vi "5.10 Occipital Lobei.vi"(9 "Randy":T3, 10 "Larry":T3) -> ()   [LabVIEW 2010]
uses:
  4-High Neurons/4.0-Timing Badass.ctl
  <vilib>/userDefined/High Color/IMAQdx.ctl
  5.10 Algorithm Parameters and Controls.ctl
  4-High Neurons/4.1.2-Act Neuron TD.ctl
  5.0-Global.vi
  <vilib>/vision/driver/NI_Vision_Acquisition_Software.lvlib
panel:
  in  "stop":bool
  out "Randy Steer Angle":dbl
  out "Larry Steer Angle":dbl
  out "Randy Certainty":dbl
  out "Larry Certainty":dbl
  in  "Rotation of Camera":dbl[][](array[numeric])=[[1.0, 0.0, 0.0], [0.0, 1.0, 0.0], [0.0, 0.0, 1.0]]
  in  "Location of Camera":dbl[](array[numeric])=[0.0, 0.0, 0.0]
  out "XY Graph":cluster{dbl[], dbl[]}[](graph)
  out "Randy Blue Actual":dbl
  out "Larry Blue Actual":dbl
  in  "Larry Exposure":dbl=0.02
  in  "Randy Exposure":dbl=0.02
  out "Randy B/W Overlay (R4)":T1(plugin-control)
  out "Randy Color Overlay (R5)":T1(plugin-control)
  in  "Randy Blue Threshold":i32=120
  out "Larry Color Overlay (L5)":T1(plugin-control)
  out "Larry B/W Overlay (L4)":T1(plugin-control)
  out "Larry Re-Map (L3)":T1(plugin-control)
  out "Randy Plane (R2)":T1(plugin-control)
  out "Larry Plane (L2)":T1(plugin-control)
  out "Randy Resample (R1)":T1(plugin-control)
  out "Larry Resample (L1)":T1(plugin-control)
  out "Raw Randy (L0)":T1(plugin-control)
  in  "Larry Blue Threshold":i32=120
  in  "Gains and Parameters":T2={"Control Gain"=0.5, "Line Setpoint in Pixels"=2.0, "Low Pass Gain"=1.2, "Image Low Pass Gain"=0.2, "Line Fullness Setpoint"=0.1, "Line Fullness Std"=0.2, "Max Filter Mod"=-10.0, "Fullness dev"=0.0}
  out "Raw Larry (L0)":T1(plugin-control)
  out "Randy Re-Map (R3)":T1(plugin-control)
  out "Super Heart Beat":T4
  in  "Resample Scaling":i32=20 min=1 max=400 step=1
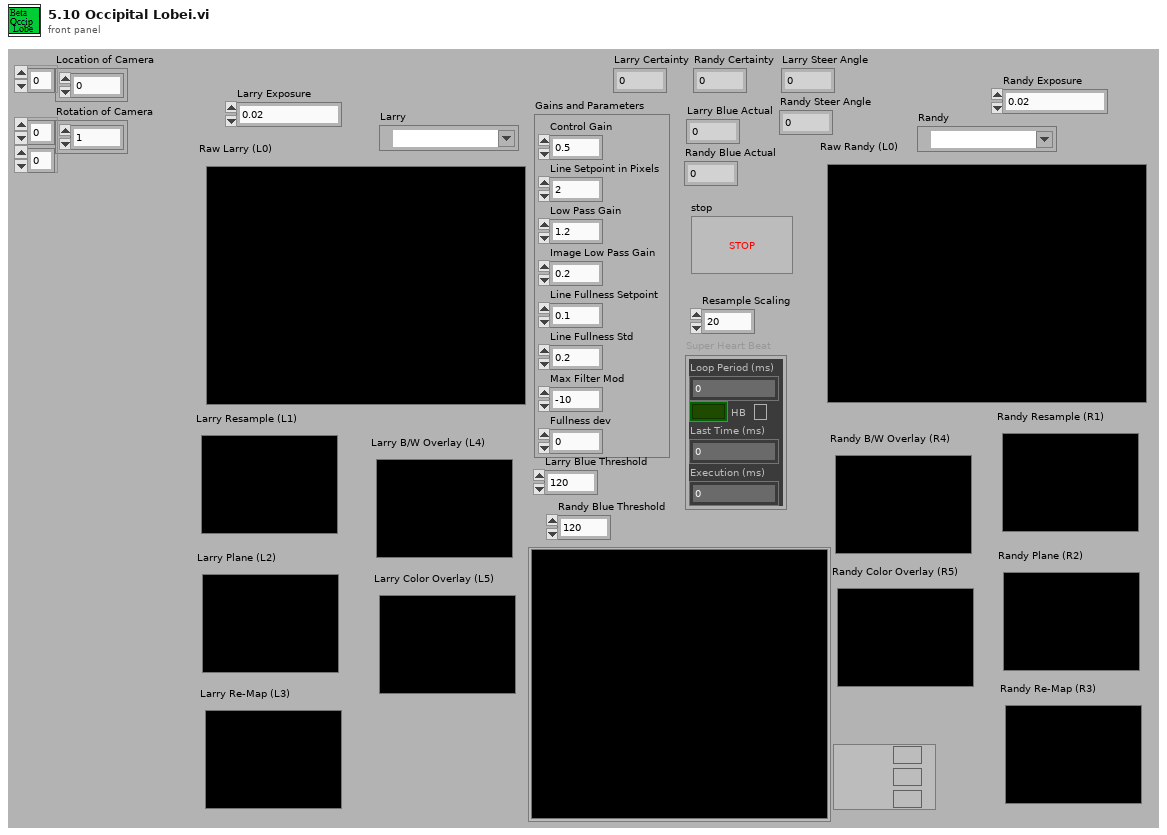
[diagram p1: front panel]
types:
  T1 = typedef "IMAQ Image.ctl" = refnum<image>
  T2 = typedef "5.10 Algorithm Parameters and Controls.ctl" = cluster{"Control Gain":dbl, "Line Setpoint in Pixels":dbl, "Low Pass Gain":dbl, "Image Low Pass Gain":dbl, "Line Fullness Setpoint":dbl, "Line Fullness Std":dbl, "Max Filter Mod":dbl, "Fullness dev":dbl}
  T3 = typedef "IMAQdx.ctl" = refnum<k21>
  T4 = typedef "4.0-Timing Badass.ctl" = cluster{"Loop Period (ms)":u32, "HB":bool, "Last Time (ms)":u32, "Execution (ms)":u32}
  T5 = typedef "5.10 Buffers Cluster.ctl" = cluster{"IMAQ Session":T3, "Buffer 0: Raw":T1, "Buffer 1: Resample":T1, "Buffer 2: Plane Extraction":T1, "Buffer 3: Re-mapping":T1, "Buffer 4: Overlay B/W":T1, "Buffer 5: Overlay Color":T1, "Buffer 6: Mask":T1, "Buffer 7: Masked Resample":T1}
  T6 = enum16{"Set Hypothalamus", "Read Hypothalamus", "Set Waypoint Arb", "Read Waypoint Arb", "Set Arb", "Read Arb", "Set Beta Occipital", "Read Beta Occipital"}
  T7 = typedef "4.1.2-Act Neuron TD.ctl" = cluster{"Speed By Path":sgl[]}
  T8 = typedef "6.10.1 LineDef.ctl" = cluster{"Vector 1 X":dbl, "Vector 1 Y":dbl, "Vector 2 X":dbl, "Vector 2 Y":dbl, "Center X":dbl, "Center Y":dbl}
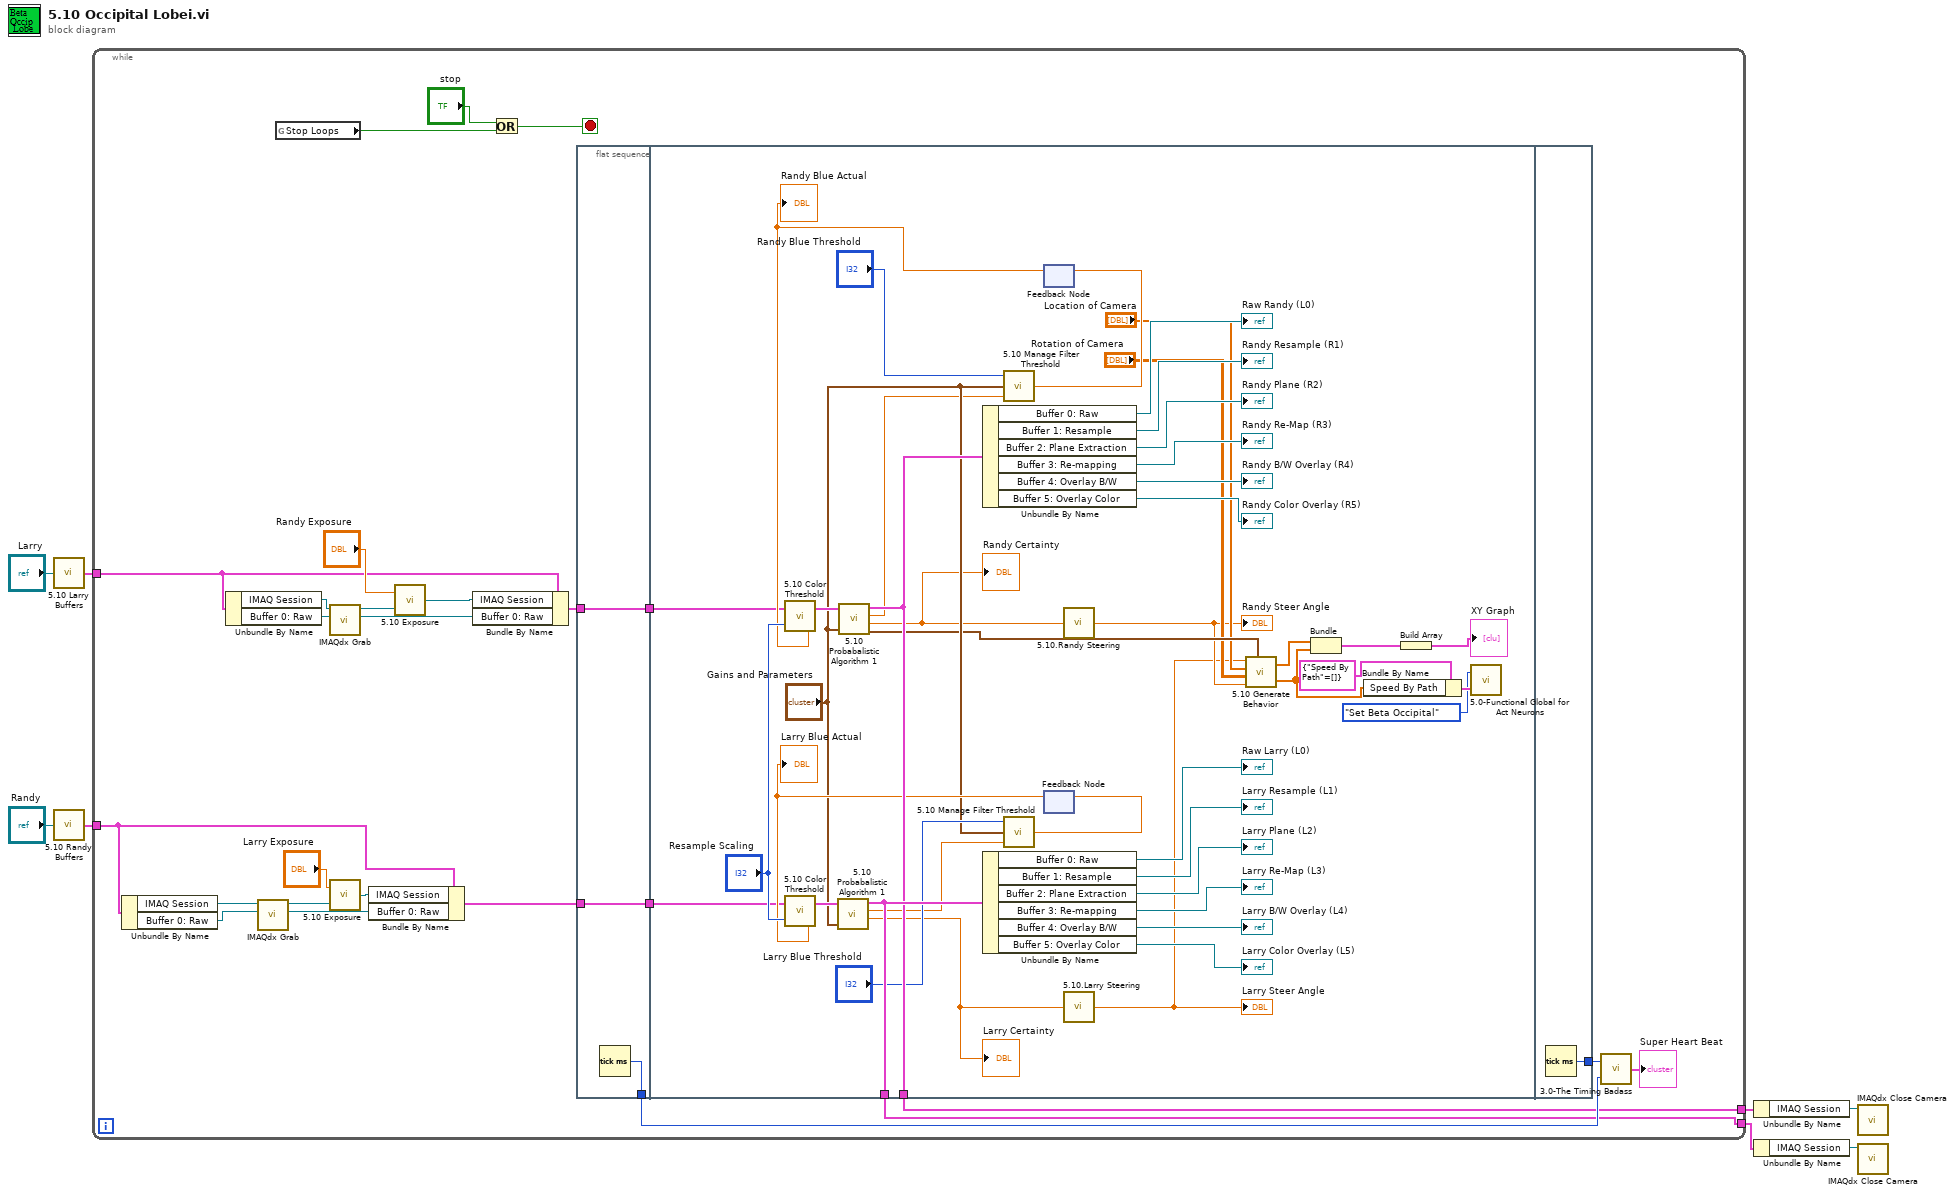
[diagram p0: block diagram]
diagram:
  n1 = call "5.10 Larry Buffers.vi"("Larry"="Larry") -> ("Larry Buffers"=w2:T5)
  n2 = call "5.10 Randy Buffers.vi"("Randy"="Randy") -> ("Randy Buffers"=w6:T5)
  n3 = while {
    tunnel: w6 -> [w13]
    tunnel: [w31] -> w5
    tunnel: w2 -> [w20]
    tunnel: [w30] -> w1
    stop <- w27 stop-if-true
    n4 = Unbundle By Name(w13) -> ("IMAQ Session"=w14:T3, "Buffer 0: Raw"=w15:T1)
    n5 = Unbundle By Name(w20) -> ("IMAQ Session"=w23:T3, "Buffer 0: Raw"=w22:T1)
    n6 = call <vilib>:"IMAQdx Grab.vi"("Image In"=w15, "Session In"=w14) -> ("Image Out"=w16:T1, "Session Out"=w17:T3)  [unwired: 6 in, 2 out]
    n7 = global read "5.0-Global.vi" "Stop Loops"() -> (w29:bool)
    n8 = call <vilib>:"IMAQdx Grab.vi"("Image In"=w22, "Session In"=w23) -> ("Image Out"=w21:T1, "Session Out"=w26:T3)  [unwired: 6 in, 2 out]
    n9 = call "5.10 Exposure.vi"("Session In"=w17, "Exposure"="Larry Exposure") -> ("Session Out"=w18:T3)
    n10 = Bundle By Name(cluster=w13, "IMAQ Session"=w18, "Buffer 0: Raw"=w16) -> (w9:T5)
    n11 = call "5.10 Exposure.vi"("Session In"=w26, "Exposure"="Randy Exposure") -> ("Session Out"=w25:T3)
    n12 = Bundle By Name(cluster=w20, "IMAQ Session"=w25, "Buffer 0: Raw"=w21) -> (w11:T5)
    n13 = Or(x="stop", y=w29) -> (x .or. y?=w27:bool)
    n14 = flat-sequence {
      tunnel: [w37] -> w33
      tunnel: [w36] -> w12
      tunnel: w11 -> [w36]
      tunnel: [w35] -> w10
      tunnel: w9 -> [w35]
      tunnel: [w77] -> w31
      tunnel: [w75] -> w30
      tunnel: w12 -> [w39]
      tunnel: w10 -> [w38]
      tunnel: [w80] -> w34
      frame #0 {
        n15 = Tick Count (ms)() -> (millisecond timer value=w37:u32)
      }
      frame #1 {
        n16 = feedback #1() -> (w54:dbl)  [unwired: 1 in]
        "Randy Blue Actual" <- w54
        n17 = call "5.10 Color Threshold.vi"("Input Fuzzy Blue Threshold"=w54, "Resample Scaling"="Resample Scaling", "Buffers In"=w39) -> ("Buffers Out"=w76:T5)
        n18 = call "5.10 Probabalistic Algorithm 1.vi"("Gains and Parameters"="Gains and Parameters", "Buffers Cluster In"=w76) -> ("Line Def"=w53:T8, "Certainty of Line (High is more certain scale is arbitrary)"=w47:dbl, "Output Control Signal"=w56:dbl, "Buffers Cluster Out"=w75:T5)  [unwired: 1 in]
        "Randy Certainty" <- w47
        n19 = Unbundle By Name(w75) -> ("Buffer 0: Raw"=→"Raw Randy (L0)":T1, "Buffer 1: Resample"=→"Randy Resample (R1)":T1, "Buffer 2: Plane Extraction"=→"Randy Plane (R2)":T1, "Buffer 3: Re-mapping"=→"Randy Re-Map (R3)":T1, "Buffer 4: Overlay B/W"=→"Randy B/W Overlay (R4)":T1, "Buffer 5: Overlay Color"=→"Randy Color Overlay (R5)":T1)
        n20 = call "5.10 Manage Filter Threshold.vi"("Output Control Signal"=w56, "Gains and Parameters"="Gains and Parameters", "Filter Control"="Randy Blue Threshold") -> ("Filter Value Output"=w55:dbl)
        n21 = feedback-in #1(w55) -> ()
        n22 = feedback #2() -> (w59:dbl)  [unwired: 1 in]
        "Larry Blue Actual" <- w59
        n23 = call "5.10 Color Threshold.vi"("Input Fuzzy Blue Threshold"=w59, "Resample Scaling"="Resample Scaling", "Buffers In"=w38) -> ("Buffers Out"=w79:T5)
        n24 = call "5.10 Probabalistic Algorithm 1.vi"("Gains and Parameters"="Gains and Parameters", "Buffers Cluster In"=w79) -> ("Certainty of Line (High is more certain scale is arbitrary)"=w48:dbl, "Output Control Signal"=w61:dbl, "Buffers Cluster Out"=w77:T5)  [unwired: 1 in, 1 out]
        "Larry Certainty" <- w48
        n25 = Unbundle By Name(w77) -> ("Buffer 0: Raw"=→"Raw Larry (L0)":T1, "Buffer 1: Resample"=→"Larry Resample (L1)":T1, "Buffer 2: Plane Extraction"=→"Larry Plane (L2)":T1, "Buffer 3: Re-mapping"=→"Larry Re-Map (L3)":T1, "Buffer 4: Overlay B/W"=→"Larry B/W Overlay (L4)":T1, "Buffer 5: Overlay Color"=→"Larry Color Overlay (L5)":T1)
        n26 = call "5.10 Manage Filter Threshold.vi"("Output Control Signal"=w61, "Gains and Parameters"="Gains and Parameters", "Filter Control"="Larry Blue Threshold") -> ("Filter Value Output"=w60:dbl)
        n27 = feedback-in #2(w60) -> ()
        n28 = call "5.10.Randy Steering.vi"("Certainty of Line (High is more certain scale is arbitrary)"=w47) -> ("Numeric"=w45:dbl)
        "Randy Steer Angle" <- w45
        n29 = call "5.10.Larry Steering.vi"("Certainty of Line (High is more certain scale is arbitrary)"=w48) -> ("Numeric"=w44:dbl)
        "Larry Steer Angle" <- w44
        n30 = call "5.10 Generate Behavior.vi"("Numeric"=w44, "Location of Camera"="Location of Camera", "Rotation of Camera"="Rotation of Camera", "Numeric 2"=w45, "Line Def"=w53) -> ("Drive Angles"=w46:dbl[], "Array"=w41:dbl[])
        n31 = Bundle("Drive Angles"=w46, "Array"=w41) -> (w50:cluster{"Drive Angles":dbl[], "Array":dbl[]})  [unwired: 1 in]
        n32 = Bundle By Name(cluster=T7 {"Speed By Path"=[]} ("Input Act Neurons"), "Speed By Path"=w41) -> (w42:T7)
        n33 = Build Array(w50) -> (→"XY Graph":cluster{"Drive Angles":dbl[], "Array":dbl[]}[])
        n34 = call "5.0-Functional Global for Act Neurons.vi"("Input Act Neurons"=w42, "Mode"=T6."Set Beta Occipital") -> ()  [unwired: 1 out]
      }
      frame #2 {
        n35 = Tick Count (ms)() -> (millisecond timer value=w80:u32)
      }
    }
    n36 = call "3.0-The Timing Badass.vi"("Start"=w33, "End"=w34) -> ("Super Heart Beat"=→"Super Heart Beat":T4)
  }
  n37 = Unbundle By Name(w1) -> ("IMAQ Session"=w3:T3)
  n38 = Unbundle By Name(w5) -> ("IMAQ Session"=w4:T3)
  n39 = call <vilib>:"IMAQdx Close Camera.vi"("Session In"=w3) -> ()  [unwired: 10 in, 1 out]
  n40 = call <vilib>:"IMAQdx Close Camera.vi"("Session In"=w4) -> ()  [unwired: 10 in, 1 out]
